vi "Point to JSON Error.vi"(8 "error in (no error)":errorcluster, 11 "JSON Lexer in":refnum<class "JSON Lexer.lvclass">) -> (0 "error out":errorcluster, 3 "JSON Lexer out":refnum<class "JSON Lexer.lvclass">)   [LabVIEW 2020, in "JKI JSON Serialization.lvlib" / "JSON Lexer.lvclass"]
doc: "Point to location of JSON parse error if possible."
uses:
  JSON Lexer.lvclass
  JSON Lexer.lvclass/JSON Lexer.ctl
  <vilib>/addons/_JKI.lib/Unicode/UTF-8 String/UTF-8 String.lvclass/UTF-8 String.ctl
  <vilib>/regexp/Match Regular Expression.xnode
  <vilib>/addons/_JKI.lib/Unicode/UTF-8 String/UTF-8 String.lvclass
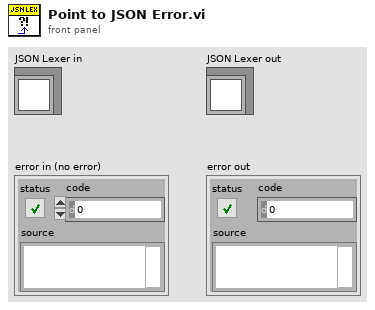
[diagram p1: front panel]
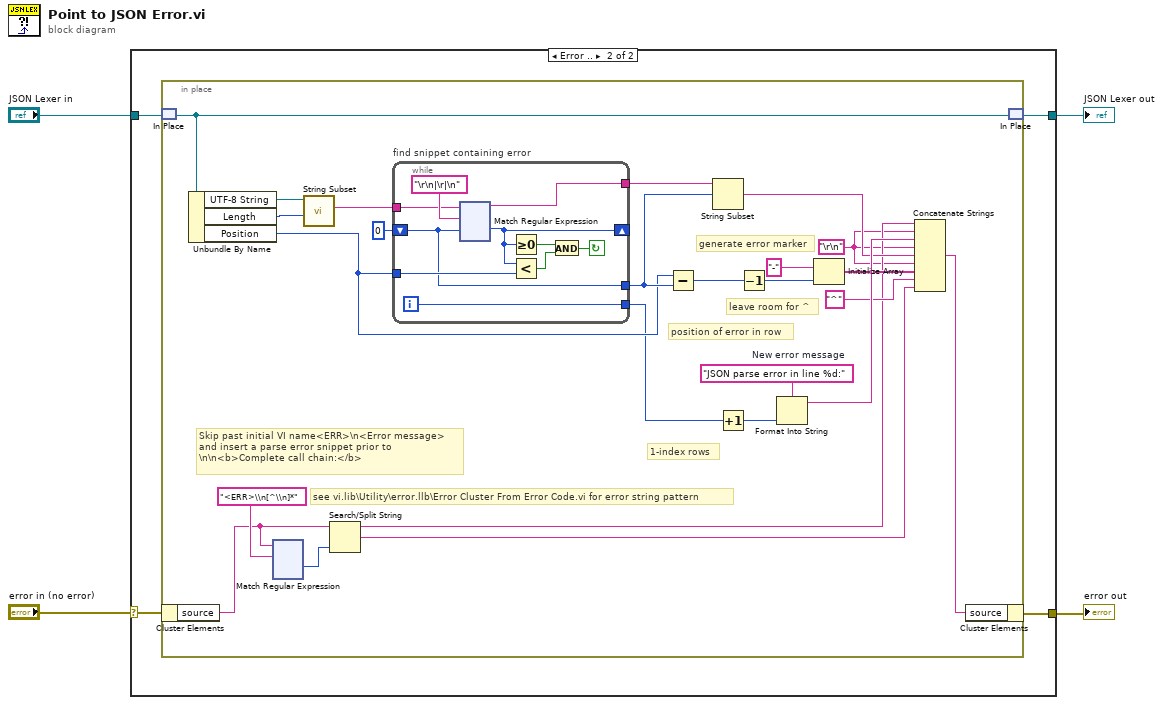
[diagram p0: block diagram]
diagram:
  n1 = case shown="Error .." "error in (no error)" {
    selector: "error in (no error)" -> [w6 w8]
    tunnel: [w5 w10] -> w4
    tunnel: "JSON Lexer in" -> [w5 w9]
    tunnel: [w6 w7] -> w1
    frame No Error {
    }
    frame Error {
      n2 = in-place {
        w29 = "JSON parse error in line %d:"  # New error message
        w14 = "\r\n"
        # "leave room for ^"
        # "see vi.lib\\Utility\\error.llb\\Error Cluster From Error Code.vi for error string pattern"
        # "Skip past initial VI name<ERR>\\n<Error message>\nand insert a parse error snippet prior to\n\\n\\n<b>Complete call chain:</b>"
        # "position of error in row"
        # "1-index rows"
        # "generate error marker"
        n3 = in-place-match #1(w9) -> (w19:refnum<class "JSON Lexer.lvclass">)
        n4 = in-place-cluster #2(w8) -> ("source"=w16:string)
        n5 = Unbundle By Name(w19) -> ("UTF-8 String"=w20:refnum<class "UTF-8 String.lvclass">, "Length"=w21:i32, "Position"=w33:i32)
        n6 = xnode "Match Regular Expression"("input string"=w16, "regular expression"="<ERR>\\n[^\\n]*") -> ("offset past match"=w17:i32)  [unwired: 4 in, 4 out]
        n7 = call <vilib>:"String Subset.vi"("Length in Bytes (0)"=w21, "UTF8 in"=w20) -> ("String Subset"=w22:string)  [unwired: 7 in, 2 out]
        n8 = Search/Split String(string=w16, offset (0)=w17) -> (substring before match=w15:string, match + rest of string=w13:string)  [unwired: 1 in, 1 out]
        n9 = while "find snippet containing error" {
          tunnel: w22 -> [w151]
          shift-right: [w150] -> _
          shift-left: 0 ("offset past replacement") -> [w152]
          tunnel: w33 -> [w157]
          tunnel: [w154] -> w24
          tunnel: [w153] -> w31
          tunnel: [w152] -> w35
          i -> [w153]
          stop <- w156 continue-if-true
          n10 = xnode "Match Regular Expression"("input string"=w151, "regular expression"="\r\n|\r|\n" ("delimiter (Tab)"), "offset (0)"=w152) -> ("before match"=w154:string, "offset past match"=w150:i32)  [unwired: 3 in, 3 out]
          n11 = Greater Or Equal To 0?(x=w150) -> (x >= 0?=w159:bool)
          n12 = Less?(x=w150, y=w157) -> (x < y?=w158:bool)
          n13 = And(x=w159, y=w158) -> (x .and. y?=w156:bool)
        }
        n14 = Subtract(x=w33, y=w35) -> (x-y=w32:i32)
        n15 = String Subset(string=w24, offset (0)=w35) -> (substring=w28:string)  [unwired: 1 in]
        n16 = Increment(x=w31) -> (x+1=w34:i32)
        n17 = Decrement(x=w32) -> (x-1=w11:i32)
        n18 = Format Into String(format string=w29, w34) -> (resulting string=w30:string)  [unwired: 2 in, 1 out]
        n19 = Initialize Array("-", w11) -> (w26:string[])
        n20 = Concatenate Strings(w15, w14, w30, w14, w28, w14, w26, "^" ("string"), w13) -> (w12:string)
        n21 = in-place-cluster #2("source"=w12) -> (w7:errorcluster)
        n22 = in-place-match #1(w19) -> (w10:refnum<class "JSON Lexer.lvclass">)
      }
    }
  }
  "error out" <- w1
  "JSON Lexer out" <- w4
